vi "PulseGenDigStart8253.vi"(0 "device":i16=1, 1 "Gate Start?":bool=TRUE, 9 "pulse delay (s)":dbl=0.1 step=0.001 format="%.6f", 11 "pulse width (s)":dbl=1.0 step=0.001 format="%.6f") -> (10 "actual delay (s)":dbl=0.001 format="%.8f", 15 "actual width (s)":dbl=0.001 format="%.8f")   [LabVIEW 2022 SP3]
doc: "DESCRIPTION:\nThis VI generates a single negative polarity pulse with a specified delay and pulse width on the OUT pin of counter 2. This delayed pulse is started with a digital line. All three counters are used for this example. Counter 0 generates the timebase, counter 1 times the delay, and counter 2 generates the delayed pulse. This VI only works with Lab/1200 type devices that have an 8253/54 counter timer chip. Examples of these devices are the PCI-1200, Lab-PC-1200, and DAQCard-1200.\n\nNOTE: This example will not work properly on the DAQCard-500 and 516 devices, which do not have a OUT0 pin.\n\n\nINSTRUCTIONS:\n1. Enter the device number of your board.\n2. Enter the digital channel and digital line.\n3. Enter the pulse delay and pulse width in seconds.\n4. Make the appropriate I/O connections as explained below.\n5. Run the VI. The negative polarity delayed pulse will be generated on the OUTB2 pin. The actual delay and actual width outputs may vary from your chosen values for reasons explained below.\n\nKEY PARAMETERS:\nThis VI shows how to use the ICTR Control.vi to generate a negative polarity pulse. Due to the nature of the 8253/54 counter/timer chip, this example has one limitation - The delay (counter 1) and the pulse (counter 2) share the same timebase from counter 0. For this reason the timebase gets set slow enough to accommodate the larger of your chosen pulse delay or pulse width without a counter rolling over. The result is that if you choose a large delay, and a short pulse, your actual pulse may differ from what you expect because the timebase may not be fine enough to accurately represent your chosen pulse width. For example if you choose a delay of 0.5 seconds and a pulse width of 10 microseconds, your actual pulse width will be 8 microseconds. This is because choosing a delay of 0.5 seconds sets up a timebase of 8 microseconds. Note that (8 microseconds)(65535) = 0.524 seconds which is why that timebase was chosen.\n\nUsing a digital line to start the delayed pulse has two advantages: The first is that you can easily modify this example to control when the digital line is set which means you can control when the pulse starts. The second is that since the delay (counter 1) is gated digitally, counter setup mode 1 (rather than mode 0) is used which has no software dependency.\n\nI/O CONNECTIONS:\nConnect your chosen digital line to GATB1 (this starts the delay).\nConnect OUTB0 to CLKB1 and CLKB2 (counter 0 generates the time base clock).\nConnect OUTB1 to GATB2 (counter 1 times the delay and gates counter 2).\nConnect to OUTB2 for the negative polarity delayed pulse.\n\nTo find the actual pin numbers, refer to the hardware user manual.\n\nDAQ VIs USED:\nICTR Control.vi"
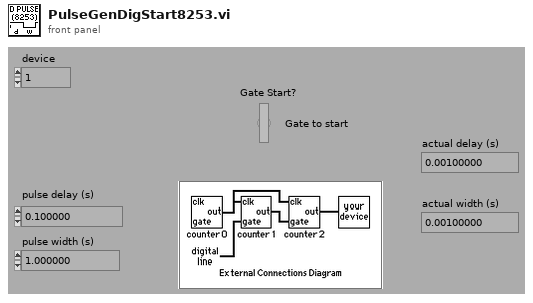
[diagram p1: front panel]
types:
  T1 = enum16{"setup mode 0", "setup mode 1", "setup mode 2", "setup mode 3", "setup mode 4", "setup mode 5", "read", "reset"}
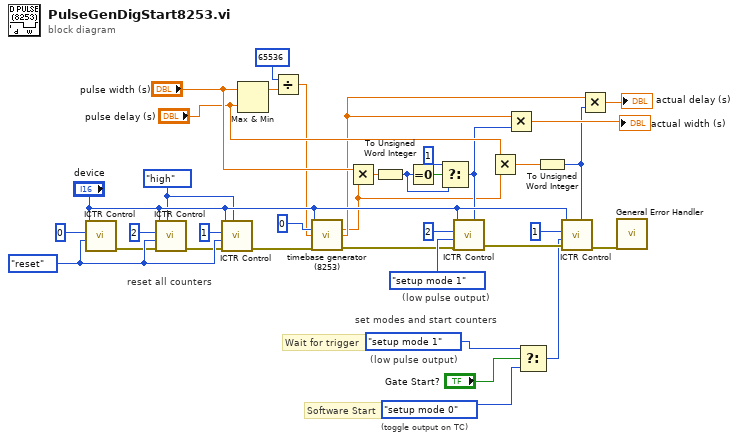
[diagram p0: block diagram]
diagram:
  w7 = enum16{"low", "high"}."high" ("output state")
  w10 = T1."reset" ("control code")
  # "Software Start"
  # "Wait for trigger"
  # "(toggle output on TC)"
  # "(low pulse output)"
  # "(low pulse output)"
  # "set modes and start counters"
  # "reset all counters"
  n1 = call <vilib>:"ICTR Control.vi"("control code"=w10, "counter"=i16 0, "device"="device") -> ("error out"=w9:errorcluster)  [unwired: 7 in, 1 out]
  n2 = call <vilib>:"ICTR Control.vi"("output state"=w7, "error in (no error)"=w9, "control code"=w10, "counter"=i16 2, "device"="device") -> ("error out"=w8:errorcluster)  [unwired: 5 in, 1 out]
  n3 = call <vilib>:"ICTR Control.vi"("output state"=w7, "error in (no error)"=w8, "control code"=w10, "counter"=i16 1, "device"="device") -> ("error out"=w6:errorcluster)  [unwired: 5 in, 1 out]
  n4 = Max & Min(x="pulse width (s)", y="pulse delay (s)") -> (max(x,y)=w29:dbl)  [unwired: 1 out]
  n5 = Divide(x=65536, y=w29) -> (x/y=w5:dbl)
  n6 = call "timebase generator (8253).vi"("device"="device", "counter"=i16 0, "frequency"=w5, "error in (no error)"=w6) -> ("actual frequency"=w16:dbl, "actual period"=w17:dbl, "error out"=w27:errorcluster)  [unwired: 7 in, 2 out]
  n7 = Multiply(x="pulse width (s)", y=w16) -> (x*y=w26:dbl)
  n8 = To Unsigned Word Integer(number=w26) -> (unsigned 16bit integer=w18:u16)
  n9 = Equal To 0?(x=w18) -> (x = 0?=w21:bool)
  n10 = Select(t=u16 1 ("counter"), s=w21, f=w18) -> (s? t:f=w19:u16)
  n11 = call <vilib>:"ICTR Control.vi"("count"=w19, "error in (no error)"=w27, "control code"=T1."setup mode 1", "counter"=i16 2, "device"="device") -> ("error out"=w30:errorcluster)  [unwired: 5 in, 1 out]
  n12 = Multiply(x="pulse delay (s)", y=w16) -> (x*y=w24:dbl)
  n13 = Multiply(x=w17, y=w19) -> (x*y=→"actual width (s)":dbl)
  n14 = Select(t=T1."setup mode 1" ("control code"), s="Gate Start?", f=T1."setup mode 0" ("control code")) -> (s? t:f=w2:T1)
  n15 = To Unsigned Word Integer(number=w24) -> (unsigned 16bit integer=w22:u16)
  n16 = call <vilib>:"ICTR Control.vi"("count"=w22, "error in (no error)"=w30, "control code"=w2, "counter"=i16 1, "device"="device") -> ("error out"=w14:errorcluster)  [unwired: 5 in, 1 out]
  n17 = Multiply(x=w17, y=w22) -> (x*y=→"actual delay (s)":dbl)
  n18 = call <vilib>:"General Error Handler.vi"("error in (no error)"=w14) -> ()  [unwired: 10 in, 5 out]
